vi "setmirrorparam.vi"(1 "Automation Refnum in":refnum<k7>) -> (0 "motorref out":refnum<k7>)   [LabVIEW 2013]
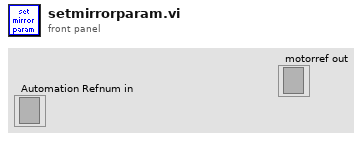
[diagram p1: front panel]
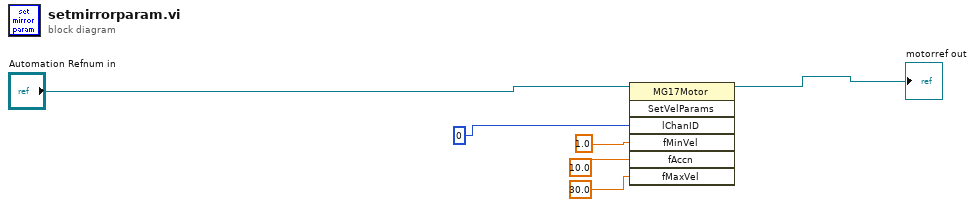
[diagram p0: block diagram]
diagram:
  n1 = invoke class="MG17Motor" method="SetVelParams"(reference="Automation Refnum in", "lChanID"=0, "fMinVel"=sgl 1.0, "fAccn"=sgl 10.0, "fMaxVel"=sgl 30.0) -> (reference out=→"motorref out":refnum<k7>)  [unwired: 2 in, 6 out]
